vi "Create And Register Generic Method Server Event.vi"(8 "error in":errorcluster, 11 "gRPCid server in":T1) -> (0 "error out":errorcluster, 2 "Generic Method Event":refnum<user-event>, 3 "gRPCid server out":T1)   [LabVIEW 2019, in "grpc-lvsupport.lvlib"]
uses:
  grpc-lvsupport.lvlib
  grpcId.ctl
  Generic Method Event Data.ctl
  <vilib>/Utility/error.llb/Error Cluster From Error Code.vi
  <resource>/labview_grpc_server.dll
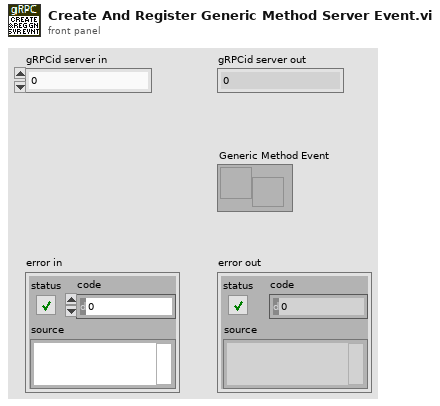
[diagram p1: front panel]
types:
  T1 = typedef "grpc-lvsupport.lvlib/grpcId.ctl" = u64
  T2 = typedef "grpc-lvsupport.lvlib/Generic Method Event Data.ctl" = cluster{"Method Name":string, "Method gRPCid":T1}
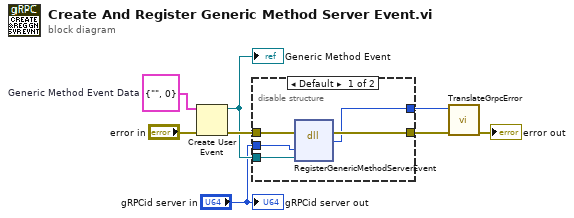
[diagram p0: block diagram]
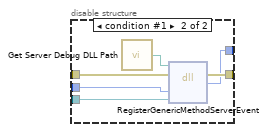
[diagram p2: hidden frame]
diagram:
  w4 = T2 {"Method Name"="", "Method gRPCid"=0}  # Generic Method Event Data
  n1 = Create User Event(user event datatype=w4, error in="error in") -> (user event=w5:refnum<user-event>, error out=w7:errorcluster)
  "Generic Method Event" <- w5
  n2 = disable-structure shown="Default" {
    disable-tunnel: w7 -> [w13 w19]
    disable-tunnel: [w12 w18] -> w6
    disable-tunnel: w5 -> [w11 w17]
    disable-tunnel: "gRPCid server in" -> [w10 w16]
    disable-tunnel: [w9 w14] -> w2
    frame condition #0 (active) {
      n3 = dll-call lib="C:/Program Files (x86)/National Instruments/LabVIEW 2024/resource/labview_grpc_server.*" fn="RegisterGenericMethodServerEvent"(error in=w13, "serverId"=w10, "genericMethodEvent"=w11) -> (error out=w12:errorcluster, "return type"=w9:i32)  [unwired: 4 in, 1 out]
    }
    frame condition #1 {
      n4 = call "Get Server Debug DLL Path.vi"() -> ("DLL Path"=w15:path)
      n5 = dll-call lib="?" fn="RegisterGenericMethodServerEvent"(path in=w15, error in=w19, "serverId"=w16, "genericMethodEvent"=w17) -> (error out=w18:errorcluster, "return type"=w14:i32)  [unwired: 3 in, 1 out]
    }
  }
  n6 = call "TranslateGrpcError.vi"("error in"=w6, "Error Code"=w2) -> ("error out"=→"error out":errorcluster)  [unwired: 9 in]
  "gRPCid server out" <- "gRPCid server in"
